vi "ReleaseQueue.vi"(7 "Force Destroy? (F)":bool, 8 "error in":errorcluster, 11 "PriorityMessageQueue in":refnum<class "PriorityMessageQueue.lvclass">) -> (0 "error out":errorcluster, 2 "Remaining Elements":refnum<class "Message.lvclass">[](array[class]))   [LabVIEW 2009, in "LapDog.Messaging.v2.lvlib" / "PriorityMessageQueue.lvclass"]
doc: "<b>This class is deprecated in version 2.1 and will be removed in version 3.0</b>\n\nThis vi runs normally even if an error occurs before this vi."
uses:
  PriorityMessageQueue.lvclass
  MessageObject/Message.lvclass
  PriorityMessageQueue.lvclass/PriorityMessageQueue.ctl
panel:
  out "Queue Name":string
  # "Queue Name output is disconnected from the connector pane while I decide how to best implement a named priority queue."
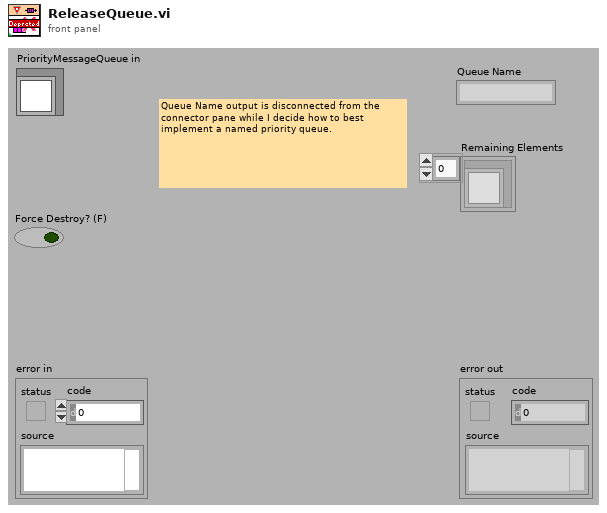
[diagram p1: front panel]
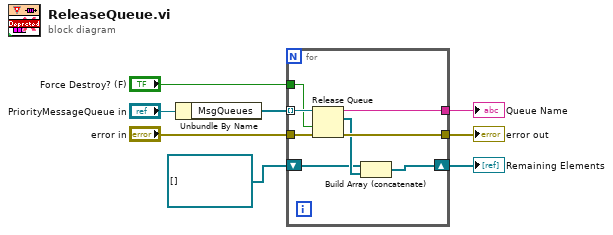
[diagram p0: block diagram]
diagram:
  n1 = Unbundle By Name("PriorityMessageQueue in") -> ("MsgQueues"=w7:refnum<queue>[])
  n2 = for {
    tunnel: w7 -> [w16] mode=indexing
    tunnel: "error in" -> [w15]
    tunnel: [w14] -> w5
    tunnel: "Force Destroy? (F)" -> [w13]
    tunnel: [w12] -> w3
    shift-right: [w10] -> w1
    shift-left: refnum<class "Message.lvclass">[] [] -> [w9]
    n3 = Release Queue(queue=w16, force destroy? (F)=w13, error in (no error)=w15) -> (queue name=w12:string, remaining elements=w11:refnum<class "Message.lvclass">[], error out=w14:errorcluster)
    n4 = Build Array (concatenate)(w9, w11) -> (w10:refnum<class "Message.lvclass">[])
  }
  "error out" <- w5
  "Remaining Elements" <- w1
  "Queue Name" <- w3
